vi "良率计算.vi"(8 "error in (no error)":errorcluster caption="错误输入（无错误）", 9 "总数输入":dbl, 10 "OK":bool, 11 "OK输入":dbl) -> (0 "error out":errorcluster caption="错误输出", 1 "良率":dbl, 2 "总数输出":dbl, 3 "OK输出":dbl)   [LabVIEW 2018]
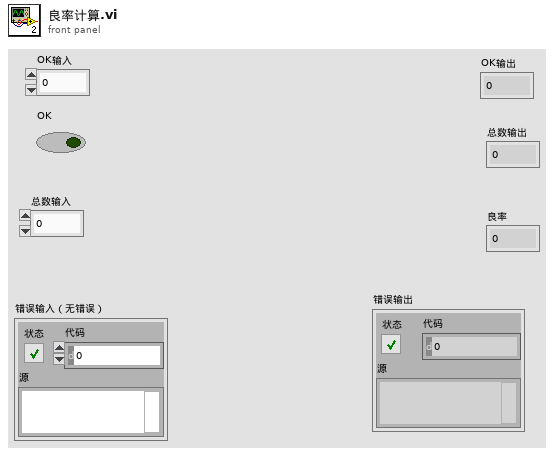
[diagram p1: front panel]
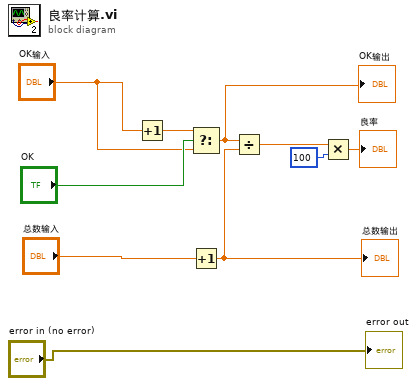
[diagram p0: block diagram]
diagram:
  n1 = Increment(x="OK输入") -> (x+1=w10:dbl)
  n2 = Select(t=w10, s="OK", f="OK输入") -> (s? t:f=w7:dbl)
  "OK输出" <- w7
  n3 = Increment(x="总数输入") -> (x+1=w6:dbl)
  "总数输出" <- w6
  n4 = Divide(x=w7, y=w6) -> (x/y=w4:dbl)
  n5 = Multiply(x=w4, y=100) -> (x*y=→"良率":dbl)
  "error out" <- "error in (no error)"
